vi "cmdtest.vi"() -> ()   [LabVIEW 2024]
panel:
  out "error out":errorcluster
  out "concatenated string":string
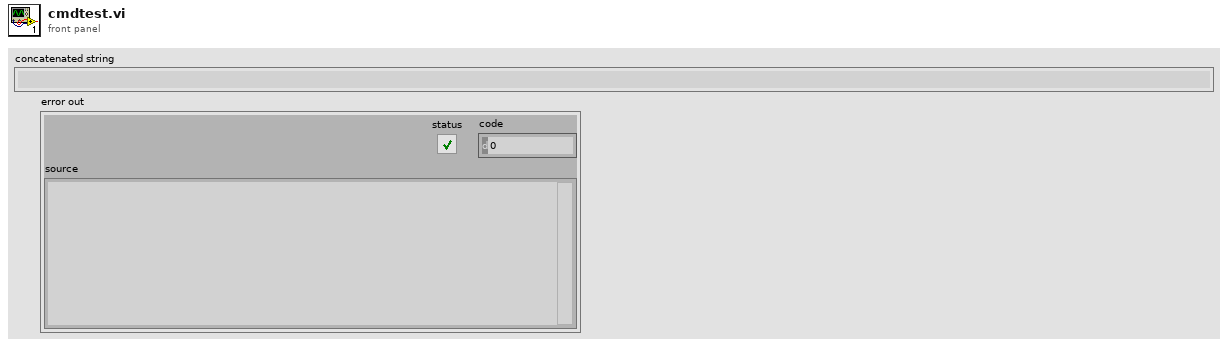
[diagram p1: front panel]
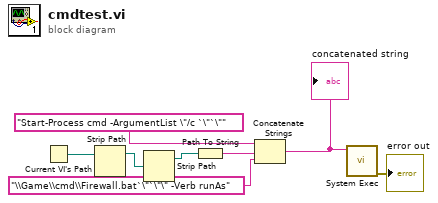
[diagram p0: block diagram]
diagram:
  n1 = Current VI's Path() -> (path=w7:path)
  n2 = Strip Path(path=w7) -> (stripped path=w2:path)  [unwired: 1 out]
  n3 = Strip Path(path=w2) -> (stripped path=w1:path)  [unwired: 1 out]
  n4 = Path To String(path=w1) -> (string=w6:string)
  n5 = Concatenate Strings("Start-Process cmd -ArgumentList \"/c `\"`\"" ("command line"), w6, "\\Game\\cmd\\Firewall.bat`\"`\"\" -Verb runAs" ("string")) -> (w3:string)
  "concatenated string" <- w3
  n6 = call <vilib>:"System Exec.vi"("command line"=w3) -> ("error out"=→"error out":errorcluster)  [unwired: 7 in, 3 out]
